vi "testTTL_htsp(broken).vi"() -> ()   [LabVIEW 2015]
uses:
  <vilib>/Platform/TimedLoop/XDataNode/timing_clust.ctl
  <vilib>/Platform/TimedLoop/XDataNode/nitl_modes.ctl
  <vilib>/Platform/TimedLoop/XDataNode/wakeup.ctl
  <vilib>/DAQmx/write.llb/DAQmx Write (Analog DBL 1Chan 1Samp).vi
  <vilib>/DAQmx/read.llb/DAQmx Read (Counter U32 1Chan 1Samp).vi
  <vilib>/DAQmx/write.llb/DAQmx Write (Digital Bool 1Line 1Point).vi
  <vilib>/DAQmx/create/channels.llb/DAQmx Create Channel (CI-Count Edges).vi
  <vilib>/DAQmx/create/timing.llb/DAQmx Create Timing Source (Digital Edge using Counter).vi
  <vilib>/DAQmx/miscellaneous.llb/DAQmx Fill In Error Info.vi
  <vilib>/platform/TimedLoop/XDataNode/XDataNode.xnode
  Windows/System32/kernel32.dll
  <resource>/objmgr/daqmx.rc
  <vilib>/Platform/TimedLoop/XDataNode/XDNodeRunTimeDep.lvlib
panel:
  out "Iteration Duration":i64
  in  "Sampling Rate (Hz)":dbl=30000.0
  out "Finished Late? [i-1]":bool
  out "count 3":u64
  in  "analog data":dbl format="%0.2f"
  out "AO error out":errorcluster
  in  "Delay lock":bool
  out "Counter error out":errorcluster
  out "sample count":u32
  in  "OEP sample clock in":tag="/Dev1/PFI1"
  in  "extra delay (samp)":i64
  out "Curr delay (samp)":i64(graph)
  out "max delay (samp)":i64
  out "wait time (ms)":dbl
  out "DO error out":errorcluster
  out "count 4":u64
  out "count 2":u64
  out "count 1":u64
  out "wait end to pulse gen end (ms)":dbl
  out "OEP to wait start (ms)":dbl caption="event rx to pulse gen start (ms)"
  out "time off (s)":dbl
  in  "Stop":bool
  out "level":sgl
  out "time on (s)":dbl
  out "New event":bool
  in  "event channel":u8=1 min=1 max=8
  out "ZMQ error out":errorcluster
  in  "port":u16=5557
  # "Timing"
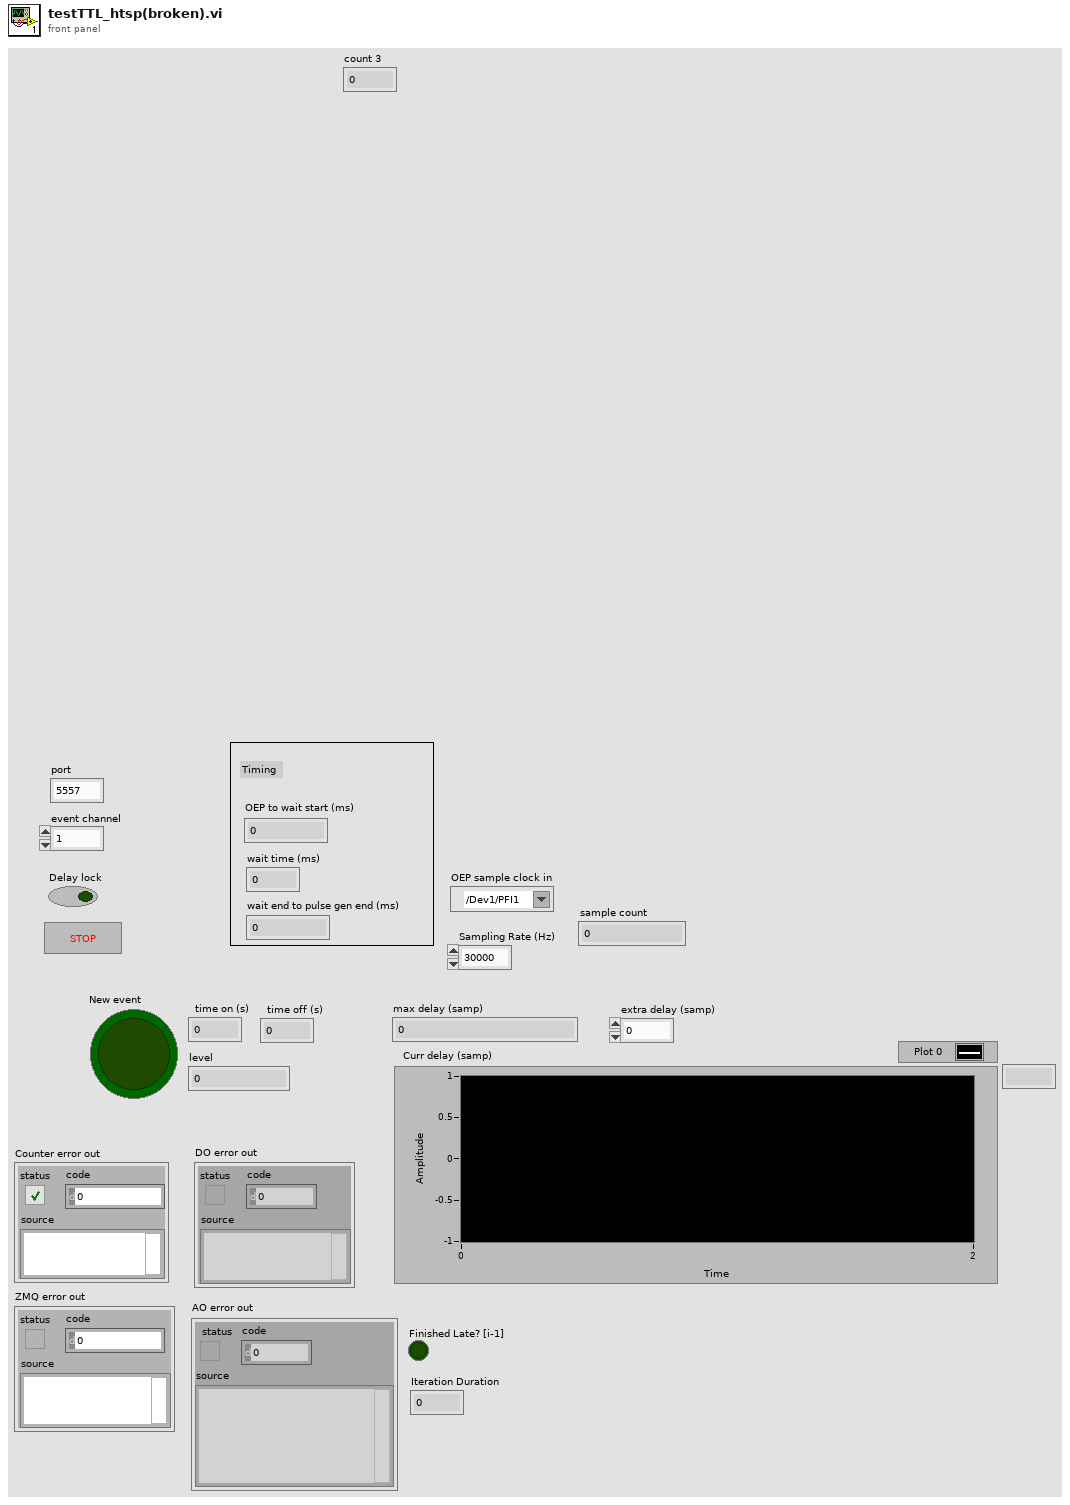
[diagram p1: front panel]
types:
  T1 = typedef "XDNodeRunTimeDep.lvlib/timing_clust.ctl" = cluster{"Expected End [f-1]":u64, "Actual End [f-1]":u64, "Finished Late? [f-1]":bool, "Expected End [i-1]":u64, "Actual End [i-1]":u64, "Finished Late? [i-1]":bool, "Expected Start [i]":u64, "Actual Start [i]":u64, "Expected Start [f]":u64, "Actual Start [f]":u64, "Source Name":string, "Structure Name":string, "Period":i64, "Deadline":i64, "Offset":i64, "Start":i64, "Priority":i32, "Timeout":i32, "Mode":T2, "Wakeup Reason":T3, "Error":errorcluster, "Source Type":string, "Secondary Source Type":string, "Global End Time":u64, "Global Start Time":u64, "Frame Duration":u64, "Iteration Duration":u64, "Assigned CPU":i32, "I/O Scan Engine Mode":u32}
  T2 = typedef "XDNodeRunTimeDep.lvlib/nitl_modes.ctl" = enum32{"No Change", "Process missed periods, maintain original phase", "Discard missed periods, maintain original phase", "Process missed periods, ignore original phase", "Discard missed periods, ignore original phase"}
  T3 = typedef "XDNodeRunTimeDep.lvlib/wakeup.ctl" = enum32{"Normal", "Aborted", "Asynchronous wakeup", "Timing source error", "Timed loop error", "Timeout"}
  T4 = enum16{"big-endian, network order", "native, host order", "little-endian"}
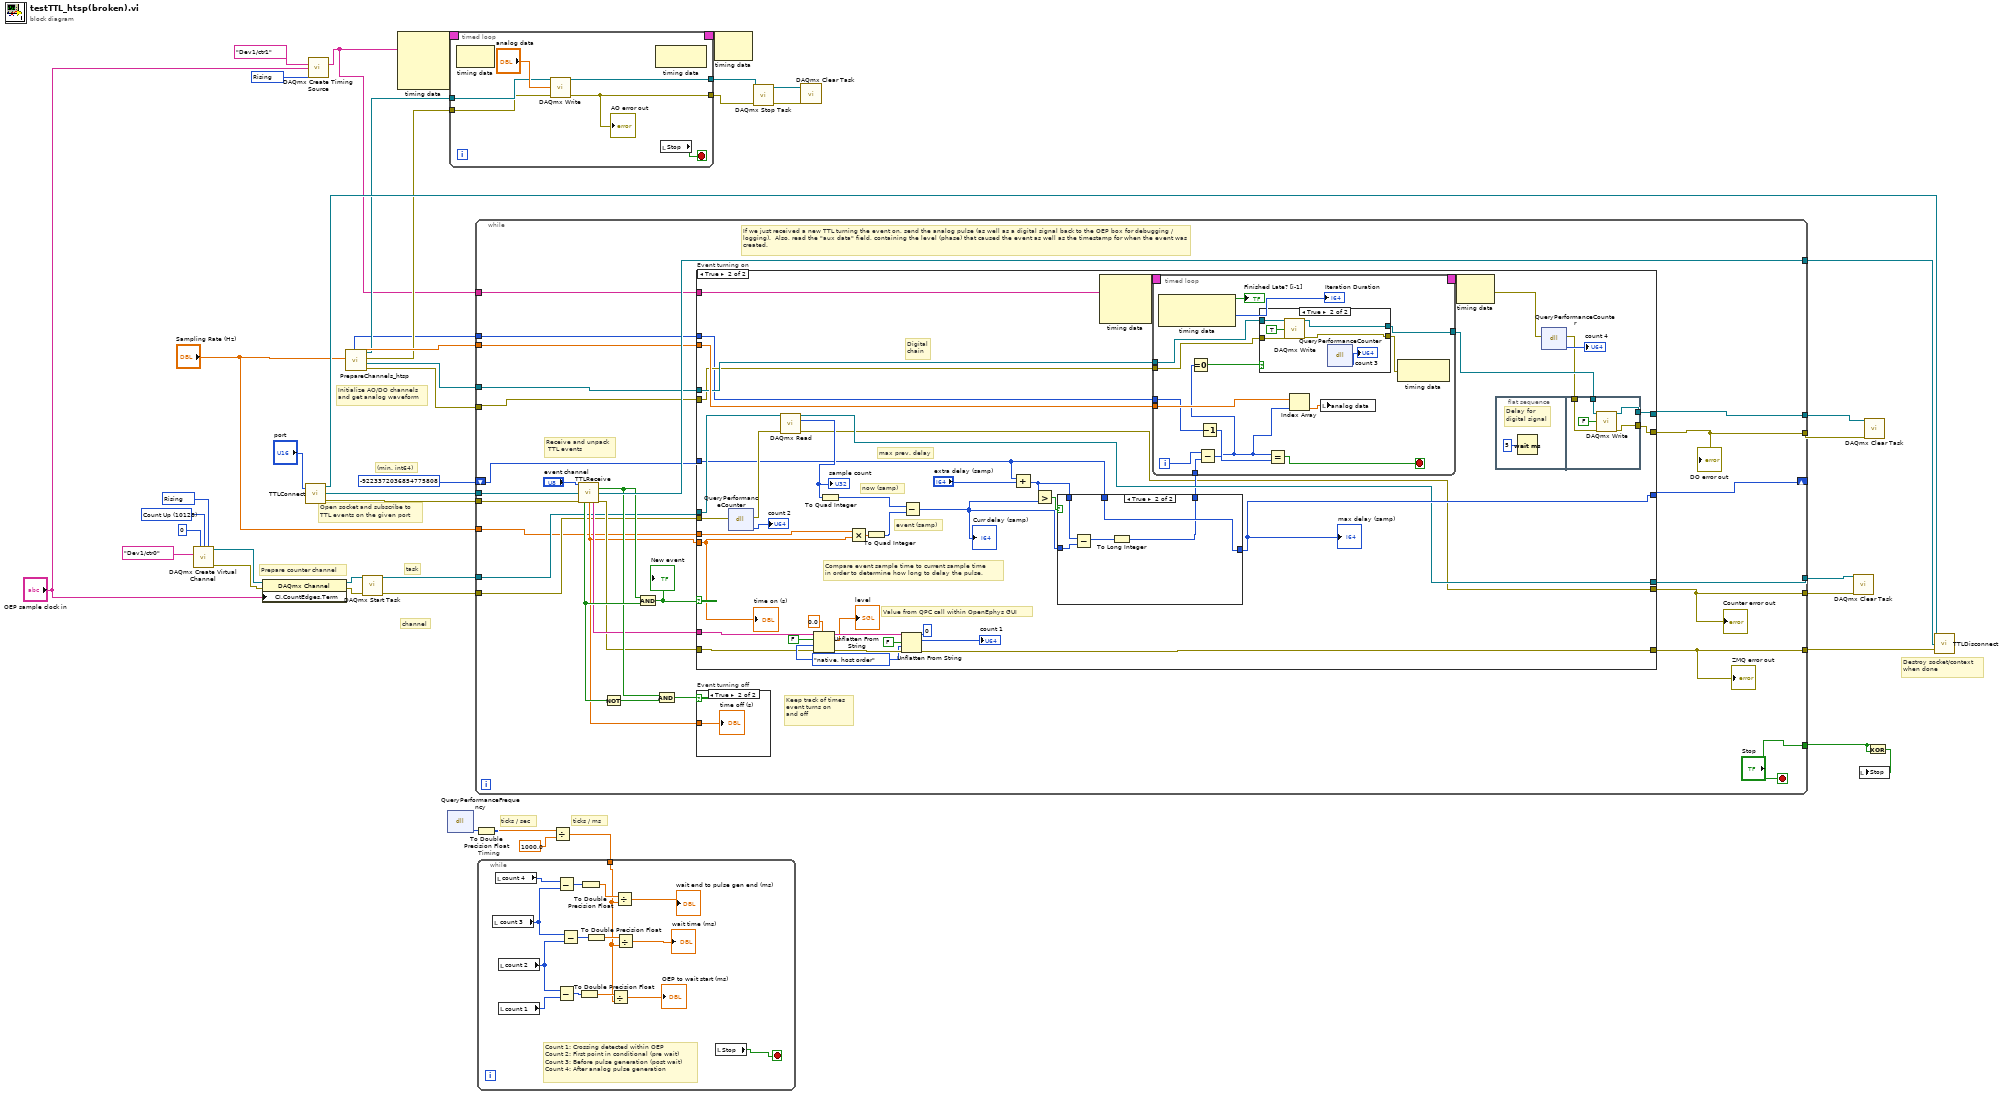
[diagram p0: block diagram]
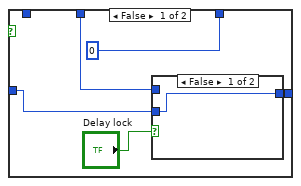
[diagram p4: hidden frame]
diagram:
  w4 = 10280 items=["Rising"=10280, "Falling"=10171] ("edge")
  w21 = 10280 items=["Rising"=10280, "Falling"=10171] ("edge")
  w22 = 10128 items=["Count Up"=10128, "Count Down"=10124, "Externally Controlled"=10326] ("count direction")
  # "channel"
  # "task"
  # "(min. int64)"
  # "Prepare counter channel"
  # "Initialize AO/DO channels\nand get analog waveform"
  # "ticks / ms"
  # "ticks / sec"
  # "Open socket and subscribe to\nTTL events on the given port"
  # "Destroy socket/context\nwhen done"
  n1 = call-poly <vilib>:"DAQmx Create Virtual Channel.vi"("initial count"=u32 0, "count direction"=w22, "edge"=w21, "counter"=tag "Dev1/ctr0") -> ("task out"=w26:refnum<k21>, "error out"=w25:errorcluster)  [unwired: 10 in]
  n2 = property class="DAQmx Channel"(reference=w26, error in=w25, "CI.CountEdges.Term"="OEP sample clock in") -> (reference out=w20:refnum<k21>, error out=w19:errorcluster)
  n3 = call "TTLConnect.vi"("port"="port") -> ("context out"=w43:refnum<class "zmq_context.lvclass">, "socket out"=w32:refnum<class "zmq_socket.lvclass">, "error out"=w33:errorcluster)  [unwired: 1 in]
  n4 = call-poly <vilib>:"DAQmx Create Timing Source.vi"("counter"=tag "Dev1/ctr1", "source"="OEP sample clock in", "edge"=w4) -> ("timing source out"=w1:string)  [unwired: 11 in, 1 out]
  n5 = call "PrepareChannels_htsp.vi"("Sampling Rate (Hz)"="Sampling Rate (Hz)") -> ("DO error out"=w40:errorcluster, "DO task out"=w41:refnum<k21>, "AO error out"=w11:errorcluster, "AO task out"=w12:refnum<k21>, "Pulse"=w13:dbl[], "Pulse length"=w7:i32)  [unwired: 5 in]
  n6 = call <vilib>:"DAQmx Start Task.vi"("task/channels in"=w20, "error in"=w19) -> ("task out"=w14:refnum<k21>, "error out"=w18:errorcluster)  [unwired: 12 in]
  n7 = node-c288(w1) -> (w6:T1)  [unwired: 3 in]
  n8 = dll-call lib="C:/Windows/System32/kernel32.dll" fn="QueryPerformanceFrequency"() -> ("lpFrequency"=w30:u64)  [unwired: 5 in, 2 out]
  n9 = timed-loop {
    tunnel: [w49] -> w9
    tunnel: [w48] -> w10
    tunnel: w12 -> [w46]
    tunnel: w11 -> [w45]
    timing: w6 -> [_]
    timing-out: [_] -> w5
    stop <- w47 stop-if-true
    n10 = node-c288() -> ()  [unwired: 1 in, 1 out]
    n11 = call-poly <vilib>:"DAQmx Write.vi"("task/channels in"=w46, "data"="analog data", "error in"=w45) -> ("task out"=w48:refnum<k21>, "error out"=w49:errorcluster)  [unwired: 10 in, 1 out]
    "AO error out" <- w49
    n12 = node-c288() -> ()  [unwired: 1 in, 1 out]
    n13 = local read "Stop"() -> (w47:bool)
  }
  n14 = while {
    tunnel: w33 -> [w80]
    tunnel: [w61] -> w31
    tunnel: [w79] -> w42
    tunnel: w32 -> [w78]
    tunnel: w41 -> [w75]
    tunnel: w40 -> [w74]
    tunnel: [w67] -> w39
    tunnel: [w62] -> w38
    tunnel: ["Stop"] -> w37
    tunnel: w13 -> [w65]
    shift-right: [w63] -> _
    shift-left: i64 -9223372036854775808 -> [w64]
    tunnel: w14 -> [w59]
    tunnel: w18 -> [w58]
    tunnel: [w57] -> w17
    tunnel: [w56] -> w16
    tunnel: "Sampling Rate (Hz)" -> [w55]
    tunnel: w7 -> [w54]
    tunnel: w1 -> [w53]
    stop <- "Stop" stop-if-true
    # "Receive and unpack\n TTL events"
    # "If we just received a new TTL turning the event on, send the analog pulse (as well as a digital signal back to the OEP box for debugging / logging).  Also, read the \"aux data\" field, containing the level (phase) that caused the event as well as the timestamp for when the event was created."
    # "Keep track of times\nevent turns on\nand off"
    n15 = call "TTLReceive.vi"("channel"="event channel", "socket in"=w78, "error in"=w80) -> ("new TTL"=w71:bool, "socket out"=w79:refnum<class "zmq_socket.lvclass">, "event on"=w72:bool, "timestamp (s)"=w60:dbl, "aux data"=w69:string, "error out"=w68:errorcluster)  [unwired: 6 in, 1 out]
    n16 = Not(x=w72) -> (.not. x?=w73:bool)
    n17 = And(x=w71, y=w72) -> (x .and. y?=w76:bool)
    "New event" <- w76
    n18 = And(x=w71, y=w73) -> (x .and. y?=w70:bool)
    n19 = case "Event turning on" shown="True" w76 {
      tunnel: w75 -> [w85 w98]
      tunnel: w74 -> [w84 w97]
      tunnel: [w85 w95] -> w67
      tunnel: [w84 w92] -> w62
      tunnel: w60 -> [_ w115]
      tunnel: w69 -> [_ w123]
      tunnel: w68 -> [w86 w121]
      tunnel: [w86 w122] -> w61
      tunnel: w65 -> [_ w99]
      tunnel: w64 -> [w83 w105]
      tunnel: [w83 w106] -> w63
      tunnel: w59 -> [w82 w117]
      tunnel: w58 -> [w81 w110]
      tunnel: [w82 w102] -> w57
      tunnel: [w81 w87] -> w56
      tunnel: w55 -> [_ w91]
      tunnel: w54 -> [_ w90]
      tunnel: w53 -> [_ w89]
      frame False {
      }
      frame True {
        w125 = T4."native, host order" ("byte order (0:big-endian, network order)")
        # "Compare event sample time to current sample time\nin order to determine how long to delay the pulse."
        # "now (samp)"
        # "event (samp)"
        # "Digital\nchain"
        # "Value from QPC call within OpenEphys GUI"
        # "max prev. delay"
        n20 = dll-call lib="C:/Windows/System32/kernel32.dll" fn="QueryPerformanceCounter" label="QPC"(error in=w110) -> (error out=w109:errorcluster, "lpPerformanceCount"=→"count 2":u64)  [unwired: 4 in, 1 out]
        n21 = call-poly <vilib>:"DAQmx Read.vi"("task/channels in"=w117, "error in"=w109) -> ("task out"=w102:refnum<k21>, "data"=w113:u32, "error out"=w87:errorcluster)  [unwired: 11 in]
        "sample count" <- w113
        n22 = Unflatten From String(type=sgl 0.0, binary string=w123, data includes array or string size? (T)=FALSE, byte order (0:big-endian, network order)=w125, error in (no error)=w121) -> (rest of the binary string=w127:string, value=→"level":sgl, error out=w128:errorcluster)
        n23 = To Quad Integer(1:w113) -> (0:w112:i64)
        n24 = Multiply(x=w91, y=w115) -> (x*y=w114:dbl)
        n25 = To Quad Integer(1:w114) -> (0:w104:i64)
        n26 = Unflatten From String(type=u64 0, binary string=w127, data includes array or string size? (T)=FALSE, byte order (0:big-endian, network order)=w125, error in (no error)=w128) -> (value=→"count 1":u64, error out=w122:errorcluster)  [unwired: 1 out]
        n27 = Subtract(x=w112, y=w104) -> (x-y=w107:i64)
        "Curr delay (samp)" <- w107
        n28 = Add(x=w105, y="extra delay (samp)") -> (x+y=w103:i64)
        n29 = Greater?(x=w103, y=w107) -> (0:w108:bool)
        n30 = case shown="True" w108 {
          tunnel: [0 w178] -> w88
          tunnel: w107 -> [w173 w181]
          tunnel: [w172 w180] -> w106
          tunnel: w105 -> [w171 w180]
          tunnel: w103 -> [_ w182]
          frame False {
            n31 = case shown="False" "Delay lock" {
              tunnel: w173 -> [w176 _]
              tunnel: [w176 w177] -> w172
              tunnel: w171 -> [_ w177]
              frame False {
              }
              frame True {
              }
            }
          }
          frame True {
            n32 = Subtract(x=w182, y=w181) -> (x-y=w179:i64)
            n33 = To Long Integer(number=w179) -> (32bit integer=w178:i32)
          }
        }
        "max delay (samp)" <- w106
        n34 = node-c288(w89) -> (w101:T1)  [unwired: 2 in]
        n35 = timed-loop {
          timing: w101 -> [_]
          timing-out: [_] -> w100
          tunnel: w99 -> [w143]
          tunnel: w98 -> [w148]
          tunnel: w97 -> [w147]
          tunnel: [w146] -> w96
          tunnel: w90 -> [w142]
          tunnel: w88 -> [w138]
          i -> [w139]
          stop <- w151 stop-if-true
          n36 = node-c288() -> (→"Finished Late? [i-1]":bool, →"Iteration Duration":i64)  [unwired: 1 in]
          n37 = Subtract(x=w139, y=w138) -> (x-y=w137:i32)
          n38 = Equal To 0?(x=w137) -> (x = 0?=w149:bool)
          n39 = Decrement(x=w142) -> (x-1=w150:i32)
          n40 = case shown="True" w149 {
            tunnel: w148 -> [w153 w157]
            tunnel: w147 -> [w152 w156]
            tunnel: [w153 w155] -> w146
            tunnel: [w152 w154] -> w145
            frame False {
            }
            frame True {
              n41 = call-poly <vilib>:"DAQmx Write.vi"("task/channels in"=w157, "data"=TRUE, "error in"=w156) -> ("task out"=w155:refnum<k21>, "error out"=w154:errorcluster)  [unwired: 10 in, 1 out]
              n42 = dll-call lib="C:/Windows/System32/kernel32.dll" fn="QueryPerformanceCounter" label="QPC"() -> ("lpPerformanceCount"=→"count 3":u64)  [unwired: 5 in, 2 out]
            }
          }
          n43 = Equal?(x=w137, y=w150) -> (x = y?=w151:bool)
          n44 = Index Array(array=w143, index=w137) -> (element=w140:dbl)
          n45 = local write "analog data"(w140) -> ()
          n46 = node-c288(w145) -> ()  [unwired: 1 out]
        }
        n47 = node-c288(w100) -> (w94:errorcluster)
        n48 = flat-sequence {
          tunnel: [w135] -> w95
          tunnel: [w134] -> w92
          tunnel: w93 -> [w133]
          tunnel: w96 -> [w132]
          frame #0 {
            # "Delay for \ndigital signal"
            n49 = Wait (ms)(milliseconds to wait=u32 5) -> ()  [unwired: 1 out]
          }
          frame #1 {
            n50 = call-poly <vilib>:"DAQmx Write.vi"("task/channels in"=w132, "data"=FALSE, "error in"=w133) -> ("task out"=w135:refnum<k21>, "error out"=w134:errorcluster)  [unwired: 10 in, 1 out]
          }
        }
        n51 = dll-call lib="C:/Windows/System32/kernel32.dll" fn="QueryPerformanceCounter" label="QPC"(error in=w94) -> (error out=w93:errorcluster, "lpPerformanceCount"=→"count 4":u64)  [unwired: 4 in, 1 out]
        "time on (s)" <- w115
      }
    }
    "DO error out" <- w62
    "ZMQ error out" <- w61
    "Counter error out" <- w56
    n52 = case "Event turning off" shown="True" w70 {
      tunnel: w60 -> [_ w183]
      frame False {
      }
      frame True {
        "time off (s)" <- w183
      }
    }
  }
  n53 = To Double Precision Float(number=w30) -> (double precision float=w28:dbl)
  n54 = Divide(x=w28, y=1000.0) -> (x/y=w27:dbl)
  n55 = while "Timing" {
    tunnel: w27 -> [w186]
    stop <- w192 stop-if-true
    # "Count 1: Crossing detected within OEP\nCount 2: First point in conditional (pre wait)\nCount 3: Before pulse generation (post wait)\nCount 4: After analog pulse generation"
    n56 = local read "count 3"() -> (w184:u64)
    n57 = local read "count 4"() -> (w198:u64)
    n58 = local read "count 2"() -> (w189:u64)
    n59 = local read "count 1"() -> (w193:u64)
    n60 = Subtract(x=w198, y=w184) -> (x-y=w197:u64)
    n61 = Subtract(x=w189, y=w193) -> (x-y=w196:u64)
    n62 = Subtract(x=w184, y=w189) -> (x-y=w188:u64)
    n63 = To Double Precision Float(number=w196) -> (double precision float=w194:dbl)
    n64 = To Double Precision Float(number=w197) -> (double precision float=w195:dbl)
    n65 = To Double Precision Float(number=w188) -> (double precision float=w187:dbl)
    n66 = Divide(x=w194, y=w186) -> (x/y=→"OEP to wait start (ms)":dbl)
    n67 = Divide(x=w195, y=w186) -> (x/y=→"wait end to pulse gen end (ms)":dbl)
    n68 = Divide(x=w187, y=w186) -> (x/y=→"wait time (ms)":dbl)
    n69 = local read "Stop"() -> (w192:bool)
  }
  n70 = node-c288(w5) -> ()  [unwired: 1 out]
  n71 = call <vilib>:"DAQmx Stop Task.vi"("task/channels in"=w10, "error in"=w9) -> ("task out"=w35:refnum<k21>, "error out"=w34:errorcluster)  [unwired: 12 in]
  n72 = call <vilib>:"DAQmx Clear Task.vi"("task in"=w35, "error in"=w34) -> ()  [unwired: 13 in, 1 out]
  n73 = call <vilib>:"DAQmx Clear Task.vi"("task in"=w17, "error in"=w16) -> ()  [unwired: 13 in, 1 out]
  n74 = call <vilib>:"DAQmx Clear Task.vi"("task in"=w39, "error in"=w38) -> ()  [unwired: 13 in, 1 out]
  n75 = Exclusive Or(1:w37, 2:w37) -> (0:w36:bool)
  n76 = local write "Stop"(w36) -> ()
  n77 = call "TTLDisconnect.vi"("error in"=w31, "socket in"=w42, "context in"=w43) -> ()  [unwired: 1 in, 1 out]
